vi "NT Write Raw.vi"(4 "options":T1={"Send All"=FALSE, "Keep Duplicates"=FALSE, "rate (hz)"=10}, 5 "description":string="raw", 6 "timestamp":u64, 8 "error in":errorcluster, 9 "value":string, 11 "name":string="Raw") -> (0 "error out":errorcluster)   [LabVIEW 2025]
doc: "Write the raw data to the named topic. This is intended for data flattened to strings. You may want to use the variant version instead."
uses:
  <vilib>/Rock Robotics/Network Tables/NT PublishOptions.ctl
  <vilib>/Rock Robotics/Network Tables/NT Datatype.ctl
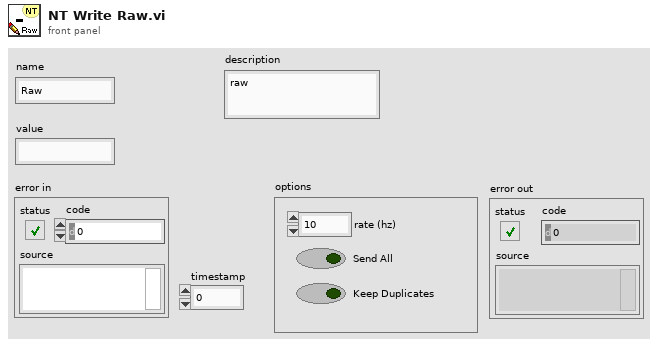
[diagram p1: front panel]
types:
  T1 = typedef "NT PublishOptions.ctl" = cluster{"Send All":bool, "Keep Duplicates":bool, "rate (hz)":u64}
  T2 = typedef "NT Datatype.ctl" = u32
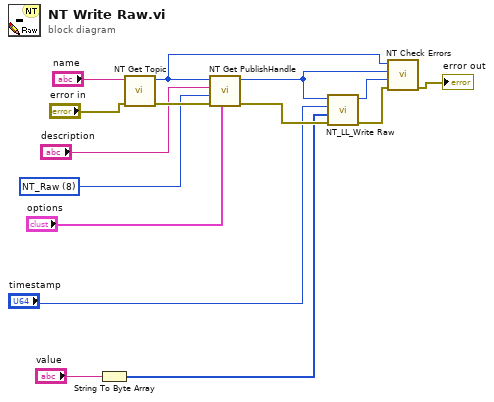
[diagram p0: block diagram]
diagram:
  w9 = T2 8 items=["NT_Unassigned"=0, "NT_Boolean"=1, "NT_Double"=2, "NT_String"=4, "NT_Raw"=8, "NT_BooleanArray"=16, "NT_DoubleArray"=32, "NT_StringArray"=64, "NT_RPC"=128, "NT_Integer"=256, "NT_Float"=512, "NT_IntegerArray"=1024, "NT_FloatArray"=2048] ("NT_Type")
  n1 = String To Byte Array(string="value") -> (unsigned byte array=w3:u8[])
  n2 = call <vilib>:"NT Get Topic.vi"("error in (no error)"="error in", "name"="name") -> ("error out"=w12:errorcluster, "topicHandle"=w6:u32)  [unwired: 8 in]
  n3 = call <vilib>:"NT Get PublishHandle.vi"("options"="options", "error in (no error)"=w12, "NT_Type"=w9, "description"="description", "topicHandle"=w6) -> ("error out"=w8:errorcluster, "publishHandle"=w5:u32)  [unwired: 5 in]
  n4 = call <vilib>:"NT_LL_Write Raw.vi"("error in (no error)"=w8, "unsigned byte array"=w3, "timestamp"="timestamp", "publishHandle"=w5) -> ("error out"=w7:errorcluster, "success"=w2:u32)  [unwired: 6 in]
  n5 = call <vilib>:"NT Check Errors.vi"("error in (no error)"=w7, "success"=w2, "pubSubHandle"=w5, "topicHandle"=w6) -> ("error out"=→"error out":errorcluster)  [unwired: 7 in]
